vi "FTW-Endpoint-Connect.vi"(0 "FTW Endpoint":refnum<class "FTW-Endpoint.lvclass">, 5 "Endpoint Address":string, 11 "error in":errorcluster) -> (4 "FTW Endpoint out":refnum<class "FTW-Endpoint.lvclass">, 15 "error out":errorcluster)   [LabVIEW 2013, in "FTW-Endpoint.lvclass"]
uses:
  FTW-Endpoint.lvclass
  FTW-Endpoint.lvclass/FTW-Endpoint.ctl
panel:
  # "Inputs"
  # "Outputs"
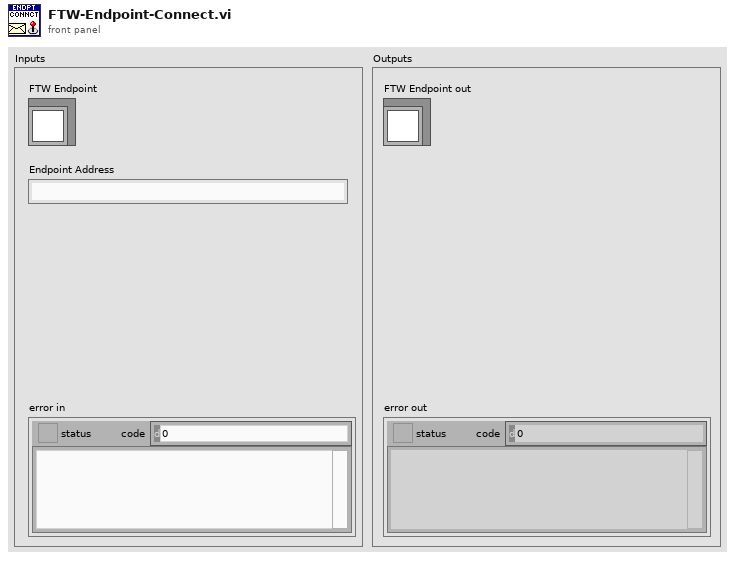
[diagram p1: front panel]
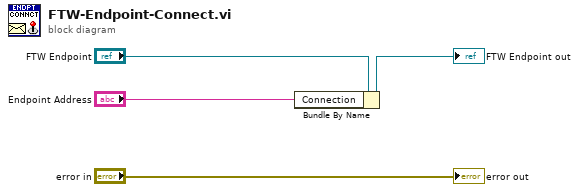
[diagram p0: block diagram]
diagram:
  n1 = Bundle By Name(cluster="FTW Endpoint", "Connection"="Endpoint Address") -> (→"FTW Endpoint out":refnum<class "FTW-Endpoint.lvclass">)
  "error out" <- "error in"
